vi "Write SQLite Connection.vi"(8 "error in (no error)":errorcluster, 10 "SQLite.lvlib:Connection":refnum<class "Connection.lvclass">, 11 "SQLite in":refnum<class "SQLite.lvclass">) -> (0 "error out":errorcluster, 3 "SQLite out":refnum<class "SQLite.lvclass">)   [LabVIEW 2021, in "SQLite.lvclass"]
uses:
  SQLite.lvclass
  <vilib>/drjdpowell/SQLite Library/SQL Connection/Connection.lvclass
  SQLite.lvclass/SQLite.ctl
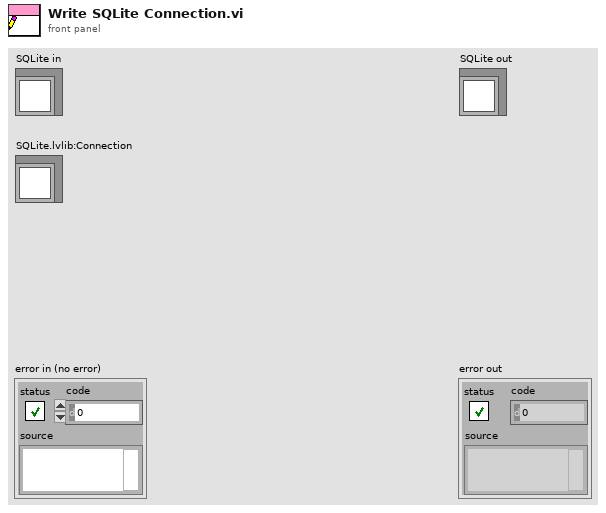
[diagram p1: front panel]
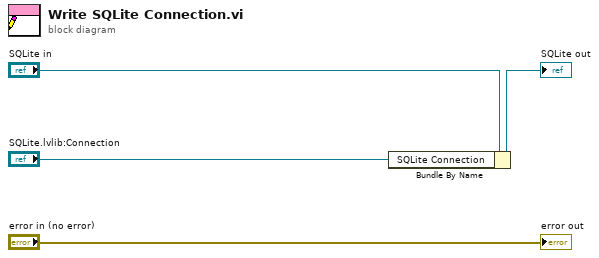
[diagram p0: block diagram]
diagram:
  n1 = Bundle By Name(cluster="SQLite in", "SQLite Connection"="SQLite.lvlib:Connection") -> (→"SQLite out":refnum<class "SQLite.lvclass">)
  "error out" <- "error in (no error)"
